vi "Miniquads.remove services.vi"(0 "i ref in":refnum<vi>, 3 "ms timeout (10000)":i32=10000, 5 "error in (no error)":errorcluster) -> (14 "i ref out":refnum<vi>, 17 "timed out":bool, 19 "error out":errorcluster)   [LabVIEW 2014, in "Miniquads.lvlib"]
doc: "Removes my DIM services."
uses:
  Miniquads.lvlib
  CSlibraries-extern/DimLVEvent/LVDimInterface/LVDimInterface.lvlib
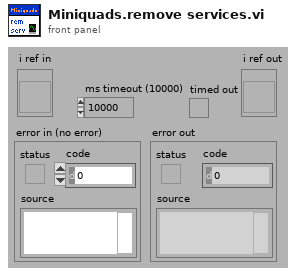
[diagram p1: front panel]
types:
  T1 = typedef "Miniquads.lvlib/Miniquads.i attribute.ctl" = cluster{"ObjectsInitialized":bool, "ObjectsLoaded":string[], "nomValues":T2, "actValues":T2}
  T2 = typedef "Miniquads.lvlib/Miniquads.voltages.ctl" = cluster{"FocusVoltage":dbl, "HorizontalVoltage":dbl, "VerticalVoltage":dbl, "serviceIDs":cluster{"FocusVoltageID":i32, "HorizontalVoltageID":i32, "VerticalVoltageID":i32}}
  T3 = cluster{"FocusVoltageID":i32, "HorizontalVoltageID":i32, "VerticalVoltageID":i32}
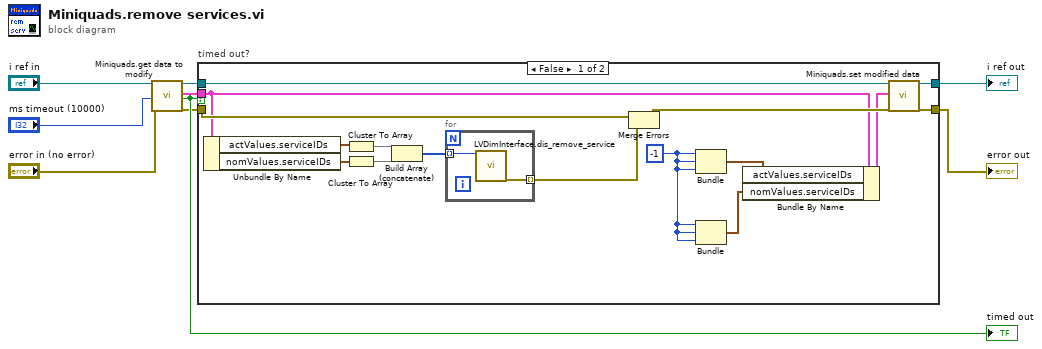
[diagram p0: block diagram]
diagram:
  n1 = call "Miniquads.get data to modify.vi"("i ref in"="i ref in", "ms timeout (10000)"="ms timeout (10000)", "error in (no error)"="error in (no error)") -> ("i ref out"=w3:refnum<vi>, "i attribute"=w1:T1, "timed out"=w4:bool, "error out"=w2:errorcluster)  [unwired: 13 in]
  "timed out" <- w4
  n2 = case "timed out?" shown="False" w4 {
    tunnel: w3 -> [w20 w29]
    tunnel: [w25 w29] -> w6
    tunnel: w2 -> [w23 w28]
    tunnel: [w24 w28] -> w8
    tunnel: w1 -> [w19 _]
    frame False {
      w10 = -1
      n3 = Unbundle By Name(w19) -> ("actValues.serviceIDs"=w12:T3, "nomValues.serviceIDs"=w11:T3)
      n4 = Cluster To Array(cluster=w12) -> (array=w18:i32[])
      n5 = Cluster To Array(cluster=w11) -> (array=w17:i32[])
      n6 = Build Array (concatenate)(w18, w17) -> (w15:i32[])
      n7 = for {
        tunnel: w15 -> [w27] mode=indexing
        tunnel: [w26] -> w14 mode=indexing
        n8 = call "LVDimInterface.dis_remove_service.vi"("my_serviceID"=w27) -> ("error out"=w26:errorcluster)  [unwired: 18 in]
      }
      n9 = Merge Errors(w23, w14) -> (w22:errorcluster)
      n10 = Bundle(w10, w10, w10) -> (w16:cluster{i32, i32, i32})  [unwired: 1 in]
      n11 = Bundle(w10, w10, w10) -> (w13:cluster{i32, i32, i32})  [unwired: 1 in]
      n12 = Bundle By Name(cluster=w19, "actValues.serviceIDs"=w16, "nomValues.serviceIDs"=w13) -> (w21:T1)
      n13 = call "Miniquads.set modified data.vi"("i ref in"=w20, "i attribute"=w21, "error in (no error)"=w22) -> ("i ref out"=w25:refnum<vi>, "error out"=w24:errorcluster)  [unwired: 15 in]
    }
    frame True {
    }
  }
  "error out" <- w8
  "i ref out" <- w6
